vi "Lvi Bridge Config Channel Settings.vi"(7 "BridgeVoltage":dbl, 8 "error in (no error)":errorcluster, 9 "BridgeConfigType":u32, 10 "Channel":u32, 11 "TaskRef":i32) -> (0 "error out":errorcluster, 2 "function return":u32(ring), 3 "TaskRef out":i32)   [LabVIEW 2022 SP3, in "DtLvLink.lvlib"]
doc: "Calls directly into the entry points of the DLL of the Data Acq SDK to configure a general-purpose bridge that returns data in voltage. If you want to return data from a bridge-based sensor in the engineering units of the sensor, use the Lvi Bridge Sensor Channel Settings VI instead."
uses:
  DtLvLink.lvlib
  <userlib>/LV-Link3/DtLvLink_64.dll
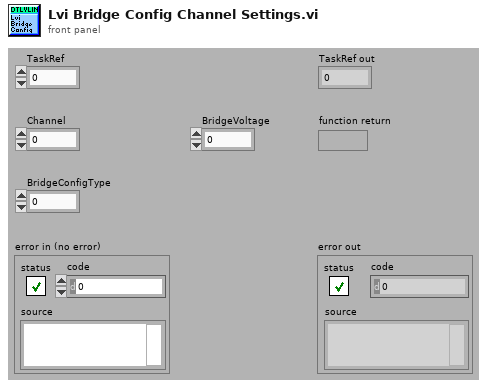
[diagram p1: front panel]
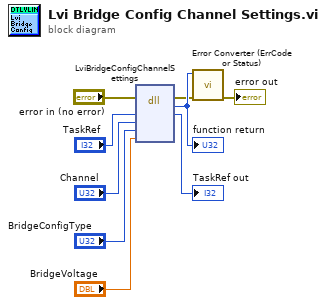
[diagram p0: block diagram]
diagram:
  n1 = dll-call lib="C:/Program Files/National Instruments/LabVIEW 2022/user.lib/LV-Link3/DtLvLink_64.*" fn="LviBridgeConfigChannelSettings"(error in="error in (no error)", "TaskRef"="TaskRef", "Channel"="Channel", "BridgeConfigType"="BridgeConfigType", "BridgeVoltage"="BridgeVoltage") -> (error out=w2:errorcluster, w9:u32, "TaskRef"=→"TaskRef out":i32)  [unwired: 5 in, 1 out]
  "function return" <- w9
  n2 = call "Error Converter (ErrCode or Status).vi"("error in (no error)"=w2, "error code"=w9) -> ("error out"=→"error out":errorcluster)  [unwired: 9 in]
